vi "录屏测试 (1).vi"() -> ()   [LabVIEW 2016]
doc: "Demonstrates how to capture the screen content with .NET functions and how to display the captured image in an IMAQ image control"
uses:
  System.Drawing
panel:
  out "录制帧率":dbl
  in  "停止":bool
  out "Image":T1(plugin-control)
  # "分辨率：1920*1080"
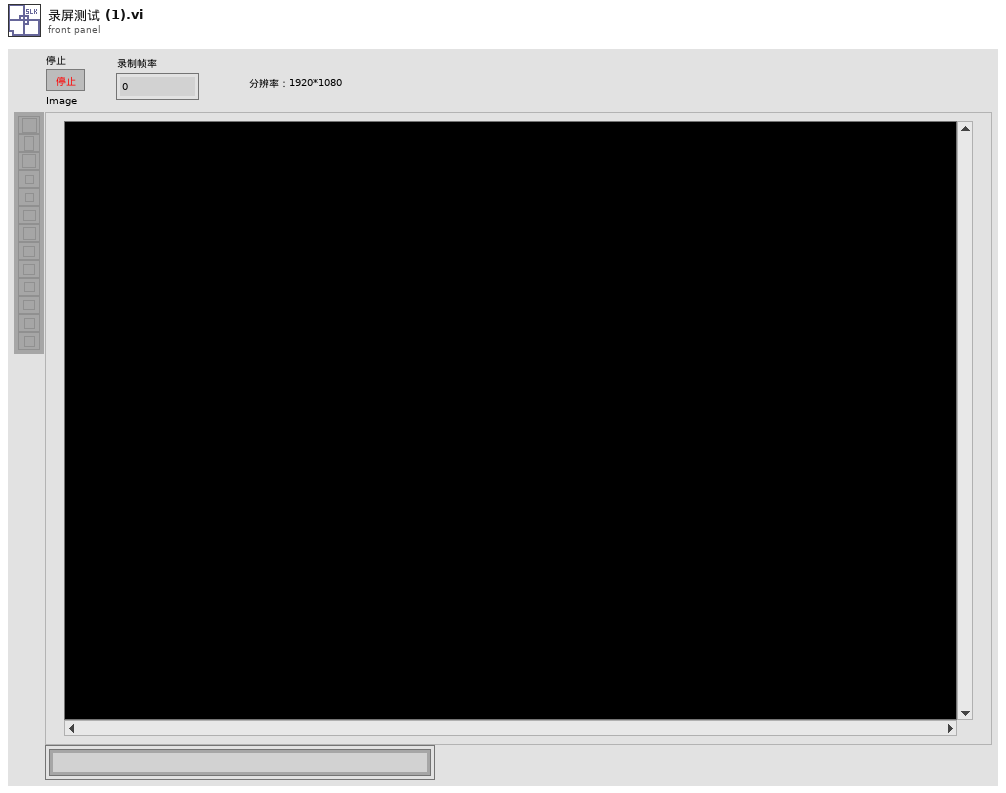
[diagram p1: front panel]
types:
  T1 = typedef "IMAQ Image.ctl" = refnum<image>
  T2 = enum32{"Map Pixel Pointer", "Unmap Pixel Pointer", "Get Pixels Infos"}
  T3 = typedef "Image Type" = u32
  T4 = typedef "LVRectTypeDef.ctl" = cluster{"Left":i16, "Top":i16, "Right":i16, "Bottom":i16}
  T5 = cluster{"Left":i32, "Top":i32, "Right":i32, "Bottom":i32}
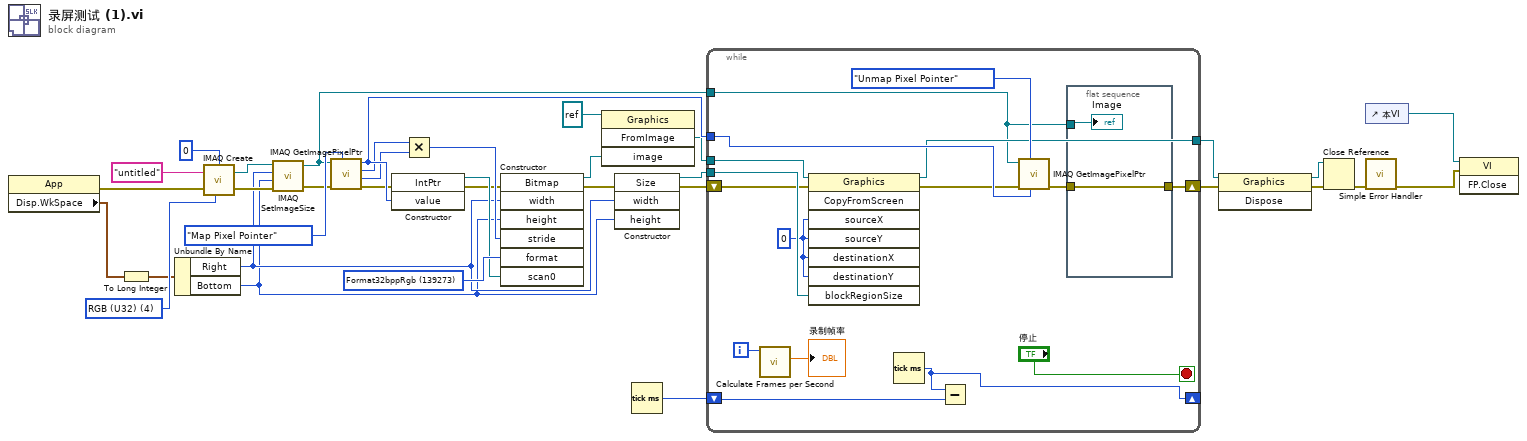
[diagram p0: block diagram]
diagram:
  w30 = 139273 items=["DontCare, Undefined"=0, "Max"=15, "Indexed"=65536, "Gdi"=131072, "Format16bppRgb555"=135173, "Format16bppRgb565"=135174, "Format24bppRgb"=137224, "Format32bppRgb"=139273, "Format1bppIndexed"=196865, "Format4bppIndexed"=197634, "Format8bppIndexed"=198659, "Alpha"=262144, "Format16bppArgb1555"=397319, "PAlpha"=524288, "Format32bppPArgb"=925707, "Extended"=1048576, "Format16bppGrayScale"=1052676, "Format48bppRgb"=1060876, "Format64bppPArgb"=1851406, "Canonical"=2097152, "Format32bppArgb"=2498570, "Format64bppArgb"=3424269] ("format")
  w32 = T3 4 items=["Grayscale (U8)", "Grayscale (I16)", "Grayscale (SGL)", "Complex (CSG)", "RGB (U32)", "HSL (U32)", "RGB (U64)", "Grayscale (U16)"] ("Image Type")
  n1 = property class="App"() -> (error out=w12:errorcluster, "Disp.WkSpace"=w24:T4)  [unwired: 2 in, 1 out]
  n2 = To Long Integer(number=w24) -> (32bit integer=w21:T5)
  n3 = Unbundle By Name(w21) -> ("Right"=w17:i32, "Bottom"=w16:i32)
  n4 = call "IMAQ Create"("Border Size"=0, "Image Name"="untitled", "Image Type"=w32, "error in (no error)"=w12) -> ("New Image"=w23:T1, "error out"=w22:errorcluster)  [unwired: 1 out]
  n5 = call "IMAQ SetImageSize"("error in (no error)"=w22, "Y Resolution"=w16, "X Resolution"=w17, "Image"=w23) -> ("error out"=w20:errorcluster, "Image Out"=w11:T1)  [unwired: 1 in]
  n6 = call "IMAQ GetImagePixelPtr"("Function"=T2."Map Pixel Pointer", "error in (no error)"=w20, "Image"=w11) -> ("error out"=w7:errorcluster, "Pixel Size (Bytes)"=w27:i32, "LineWidth(Pixels)"=w28:i32, "Pixel Pointer out"=w35:u64)  [unwired: 3 in, 2 out]
  n7 = constructor class="IntPtr"(error in=w7, "value"=w35) -> (reference out=w29:refnum<k24>, error out=w25:errorcluster)  [unwired: 2 in, 2 out]
  n8 = Multiply(x=w28, y=w27) -> (x*y=w26:i32)
  n9 = constructor class="Bitmap"(error in=w25, "width"=w17, "height"=w16, "stride"=w26, "format"=w30, "scan0"=w29) -> (reference out=w5:refnum<k24>, error out=w19:errorcluster)  [unwired: 2 in, 6 out]
  n10 = invoke class="Graphics" method="FromImage"(reference=refnum<k24> refnum, "image"=w5) -> ("FromImage"=w4:refnum<k24>)  [unwired: 2 in, 3 out]
  n11 = constructor class="Size"(error in=w19, "width"=w17, "height"=w16) -> (reference out=w18:refnum<k24>, error out=w15:errorcluster)  [unwired: 2 in, 3 out]
  n12 = Tick Count (ms)() -> (millisecond timer value=w3:u32)
  n13 = while {
    tunnel: w35 -> [w51]
    tunnel: w18 -> [w49]
    tunnel: [w46] -> w14
    tunnel: w11 -> [w38]
    shift-right: [w36] -> w8
    shift-left: w15 -> [w41]
    tunnel: w4 -> [w42]
    shift-right: [w39] -> _
    shift-left: w3 -> [w40]
    i -> [w44]
    stop <- "停止" stop-if-true
    w48 = 0 ("sourceX")
    n14 = call <vilib>:"Calculate Frames per Second.vi"("Buffer Number"=w44) -> ("Processed Frames/s"=→"录制帧率":dbl)  [unwired: 8 in, 2 out]
    n15 = invoke class="Graphics" method="CopyFromScreen"(reference=w42, error in=w41, "sourceX"=w48, "sourceY"=w48, "destinationX"=w48, "destinationY"=w48, "blockRegionSize"=w49) -> (reference out=w46:refnum<k24>, error out=w47:errorcluster)  [unwired: 1 in, 6 out]
    n16 = Tick Count (ms)() -> (millisecond timer value=w39:u32)
    n17 = Subtract(x=w39, y=w40) -> ()  [unwired: 1 out]
    n18 = call "IMAQ GetImagePixelPtr"("Pixel Pointer in"=w51, "Function"=T2."Unmap Pixel Pointer", "error in (no error)"=w47, "Image"=w38) -> ("error out"=w37:errorcluster)  [unwired: 2 in, 5 out]
    n19 = flat-sequence {
      tunnel: w38 -> [w52]
      tunnel: w37 -> [w53]
      tunnel: [w53] -> w36
      frame #0 {
        "Image" <- w52
      }
    }
  }
  n20 = invoke class="Graphics" method="Dispose"(reference=w14, error in=w8) -> (reference out=w10:refnum<k24>, error out=w13:errorcluster)  [unwired: 1 in, 1 out]
  n21 = Close Reference(reference=w10, error in (no error)=w13) -> (error out=w9:errorcluster)
  n22 = control-ref of="本VI"() -> (w2:refnum<vi>)
  n23 = call <vilib>:"Simple Error Handler.vi"("error in (no error)"=w9) -> ("error out"=w1:errorcluster)  [unwired: 4 in, 4 out]
  n24 = invoke class="VI" method="FP.Close"(reference=w2, error in=w1) -> ()  [unwired: 1 in, 3 out]
